vi "r_table_list.vi"(6 "ms timeout (0:default)":i32, 7 "db":string, 8 "error in (no error)":errorcluster, 11 "rethinkdb in":T1) -> (0 "error out":errorcluster, 2 "table list":string[](array[string]), 3 "rethinkdb out":T1)   [LabVIEW 2017, in "rethinkdb.lvlib"]
uses:
  refnum.ctl
  ql2_term.ctl
  ql2_query.ctl
  ql2_term_to_id.vi
  ql2_query_to_id.vi
  rethinkdb.lvlib
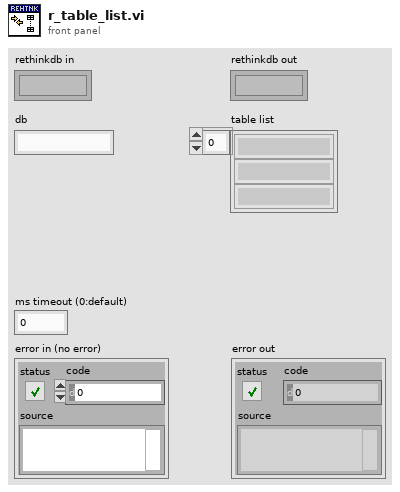
[diagram p1: front panel]
types:
  T1 = typedef "rethinkdb.lvlib/refnum.ctl" = refnum<k1>
  T2 = typedef "rethinkdb.lvlib/ql2_term.ctl" = enum8{"ADD", "AND", "APPEND", "APRIL", "ARGS", "ASC", "AUGUST", "AVG", "BETWEEN", "BETWEEN_DEPRECATED", "BINARY", "BIT_AND", "BIT_NOT", "BIT_OR", "BIT_SAL", "BIT_SAR", "BIT_XOR", "BRACKET", "BRANCH", "CEIL", "CHANGES", "CHANGE_AT", "CIRCLE", "COERCE_TO", "CONCAT_MAP", "CONFIG", "CONTAINS", "COUNT", "DATE", "DATUM", "DAY", "DAY_OF_WEEK", "DAY_OF_YEAR", "DB", "DB_CREATE", "DB_DROP", "DB_LIST", "DECEMBER", "DEFAULT", "DELETE", "DELETE_AT", "DESC", "DIFFERENCE", "DISTANCE", "DISTINCT", "DIV", "DOWNCASE", "DURING", "EPOCH_TIME", "EQ", "EQ_JOIN", "ERROR", "FEBRUARY", "FILL", "FILTER", "FLOOR", "FOLD", "FOR_EACH", "FRIDAY", "FUNC", "FUNCALL", "GE", "GEOJSON", "GET", "GET_ALL", "GET_FIELD", "GET_INTERSECTING", "GET_NEAREST", "GET_WRITE_HOOK", "GRANT", "GROUP", "GT", "HAS_FIELDS", "HOURS", "HTTP", "IMPLICIT_VAR", "INCLUDES", "INDEX_CREATE", "INDEX_DROP", "INDEX_LIST", "INDEX_RENAME", "INDEX_STATUS", "INDEX_WAIT", "INFO", "INNER_JOIN", "INSERT", "INSERT_AT", "INTERSECTS", "IN_TIMEZONE", "ISO8601", "IS_EMPTY", "JANUARY", "JAVASCRIPT", "JSON", "JULY", "JUNE", "KEYS", "LE", "LIMIT", "LINE", "LITERAL", "LT", "MAKE_ARRAY", "MAKE_OBJ", "MAP", "MARCH", "MATCH", "MAX", "MAXVAL", "MAY", "MERGE", "MIN", "MINUTES", "MINVAL", "MOD", "MONDAY", "MONTH", "MUL", "NE", "NOT", "NOVEMBER", "NOW", "NTH", "OBJECT", "OCTOBER", "OFFSETS_OF", "OR", "ORDER_BY", "OUTER_JOIN", "PLUCK", "POINT", "POLYGON", "POLYGON_SUB", "PREPEND", "RANDOM", "RANGE", "REBALANCE", "RECONFIGURE", "REDUCE", "REPLACE", "ROUND", "SAMPLE", "SATURDAY", "SECONDS", "SEPTEMBER", "SET_DIFFERENCE", "SET_INSERT", "SET_INTERSECTION", "SET_UNION", "SET_WRITE_HOOK", "SKIP", "SLICE", "SPLICE_AT", "SPLIT", "STATUS", "SUB", "SUM", "SUNDAY", "SYNC", "TABLE", "TABLE_CREATE", "TABLE_DROP", "TABLE_LIST", "THURSDAY", "TIME", "TIMEZONE", "TIME_OF_DAY", "TO_EPOCH_TIME", "TO_GEOJSON", "TO_ISO8601", "TO_JSON_STRING", "TUESDAY", "TYPE_OF", "UNGROUP", "UNION", "UPCASE", "UPDATE", "UUID", "VALUES", "VAR", "WAIT", "WEDNESDAY", "WITHOUT", "WITH_FIELDS", "YEAR", "ZIP", "invalid"}
  T3 = typedef "rethinkdb.lvlib/ql2_query.ctl" = enum8{"START", "CONTINUE", "STOP", "NOREPLY_WAIT", "SERVER_INFO", "invalid"}
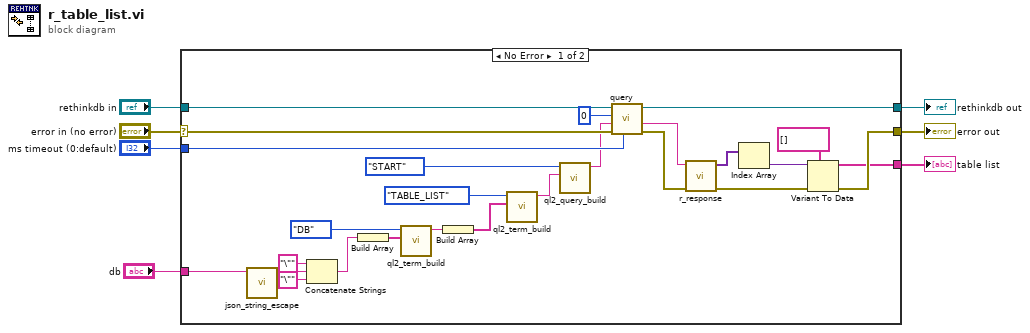
[diagram p0: block diagram]
diagram:
  n1 = case shown="No Error" "error in (no error)" {
    selector: "error in (no error)" -> [w33 w35]
    tunnel: "rethinkdb in" -> [w32 w34]
    tunnel: [w31 w34] -> w5
    tunnel: "ms timeout (0:default)" -> [w30 _]
    tunnel: [w23 w35] -> w3
    tunnel: [w20 _] -> w2
    tunnel: "db" -> [w9 _]
    frame No Error {
      n2 = call "json_string_escape.vi"("string"=w9) -> ("escaped string"=w12:string)  [unwired: 10 in]
      n3 = Concatenate Strings("\"" ("string"), w12, "\"" ("string")) -> (w8:string)
      n4 = Build Array(w8) -> (w16:string[])
      n5 = call "ql2_term_build.vi"("args"=w16, "term_type"=ql2_term."DB") -> ("query"=w15:string)  [unwired: 9 in]
      n6 = Build Array(w15) -> (w14:string[])
      n7 = call "ql2_term_build.vi"("args"=w14, "term_type"=ql2_term."TABLE_LIST") -> ("query"=w13:string)  [unwired: 9 in]
      n8 = call "ql2_query_build.vi"("query"=w13, "query_type"=ql2_query."START") -> ("query"=w28:string)  [unwired: 9 in]
      n9 = call "query.vi"("ms timeout (0:default)"=w30, "error in (no error)"=w33, "query"=w28, "token in (random)"=u64 0, "rethinkdb in"=w32) -> ("error out"=w27:errorcluster, "response"=w25:string, "rethinkdb out"=w31:T1)  [unwired: 3 in, 1 out]
      n10 = call "r_response.vi"("error in (no error)"=w27, "response"=w25) -> ("error out"=w26:errorcluster, "values"=w24:variant[])  [unwired: 8 in]
      n11 = Index Array(array=w24) -> (element=w22:variant)  [unwired: 1 in]
      n12 = Variant To Data(error in=w26, type=string[] [], Variant=w22) -> (data=w20:string[], error out=w23:errorcluster)
    }
    frame Error {
    }
  }
  "error out" <- w3
  "rethinkdb out" <- w5
  "table list" <- w2
